vi "Reconnect.vi"(8 "error in (no error)":errorcluster, 11 "navX - SPI in":refnum<class "navX - SPI.lvclass">) -> (0 "error out":errorcluster, 3 "navX - SPI out":refnum<class "navX - SPI.lvclass">)   [LabVIEW 2015, in "navX Library v3.lvlib" / "navX - SPI.lvclass"]
uses:
  navX - SPI.lvclass
  navX - SPI.lvclass/navX - SPI.ctl
  navX - Interface/navX - Interface.lvclass
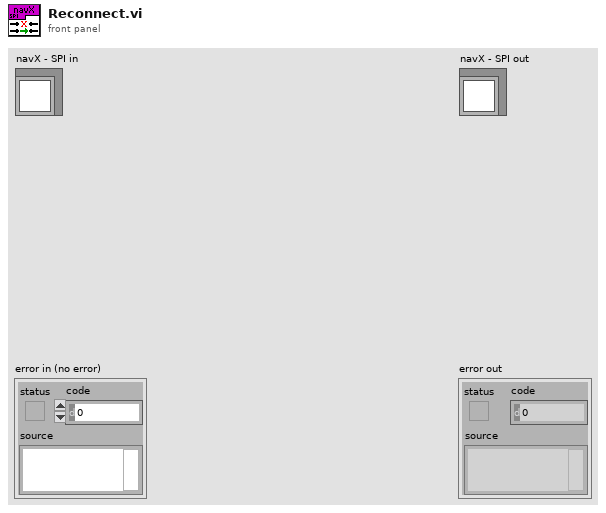
[diagram p1: front panel]
types:
  T1 = typedef "spi_bus.ctl" = enum16{"SPI On-Board, CS0", "SPI On-Board, CS1", "SPI On-Board, CS2", "SPI On-Board, CS3", "SPI MXP", "Invalid"}
  T2 = typedef "WPI_SPIDevRef.ctl" = cluster{"DevStatus":errorcluster, "Handle":i32, "SPI Bus":T1}
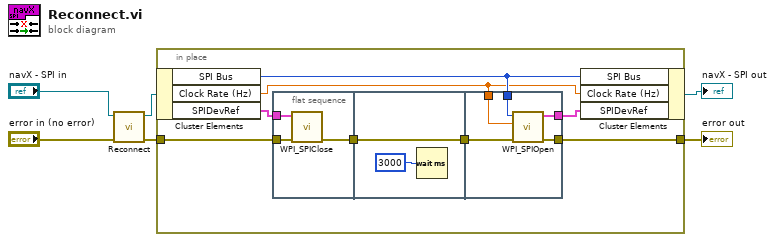
[diagram p0: block diagram]
diagram:
  n1 = call-parent "Reconnect.vi"("error in (no error)"="error in (no error)", "navX - Interface in"="navX - SPI in") -> ("error out"=w2:errorcluster, "navX - Interface out"=w4:refnum<class "navX - SPI.lvclass">)  [unwired: 8 in]
  n2 = in-place {
    in-place-border: [w14] -> w3
    in-place-border: w2 -> [w13]
    n3 = in-place-cluster #1(w4) -> ("SPI Bus"=w8:T1, "Clock Rate (Hz)"=w7:dbl, "SPIDevRef"=w12:T2)
    n4 = flat-sequence {
      tunnel: w13 -> [w16]
      tunnel: w12 -> [w17]
      tunnel: [w15] -> w10
      tunnel: w10 -> [w19]
      tunnel: [w19] -> w9
      tunnel: [w24] -> w11
      tunnel: [w23] -> w14
      tunnel: w9 -> [w20]
      tunnel: w8 -> [w22]
      tunnel: w7 -> [w21]
      frame #0 {
        n5 = call <vilib>:"WPI_SPIClose.vi"("error in (no error)"=w16, "SPIDevRef"=w17) -> ("error out"=w15:errorcluster)  [unwired: 9 in]
      }
      frame #1 {
        n6 = Wait (ms)(milliseconds to wait=u32 3000) -> ()  [unwired: 1 out]
      }
      frame #2 {
        n7 = call <vilib>:"WPI_SPIOpen.vi"("error in"=w20, "Clock Rate (Hz)"=w21, "SPI Bus"=w22) -> ("error out"=w23:errorcluster, "SPIDevRef"=w24:T2)  [unwired: 7 in]
      }
    }
    n8 = in-place-cluster #1("SPI Bus"=w8, "Clock Rate (Hz)"=w7, "SPIDevRef"=w11) -> (→"navX - SPI out":refnum<class "navX - SPI.lvclass">)
  }
  "error out" <- w3
